vi "Close.vi"(8 "error in (no error)":errorcluster, 11 "Writer in":refnum<class "Writer.lvclass">) -> (0 "error out":errorcluster)   [LabVIEW 2022 SP3, in "Enclave.lvlib" / "Writer.lvclass"]
uses:
  Writer.lvclass
  Writer.lvclass/Writer.ctl
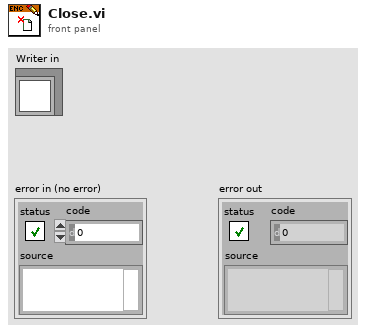
[diagram p1: front panel]
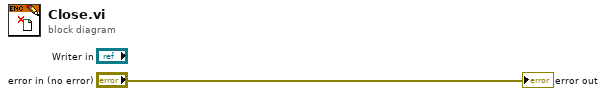
[diagram p0: block diagram]
diagram:
  "error out" <- "error in (no error)"
